vi "Arm - In Position Detector.vi"(6 "Angle Tolerance (+/-)":dbl=2.0 format="%#_13g", 8 "error in (no error)":errorcluster, 10 "Set Angle":dbl, 11 "AIDeviceRef":T1={"DevStatus"={"status"=FALSE, "code"=0, "source"=""}, "Analog Channel"=enum."Invalid"}) -> (0 "error out":errorcluster, 1 "In Position":bool, 2 "Current Angle":dbl, 4 "LED Control (Blink / On)":bool)   [LabVIEW 2015]
uses:
  <vilib>/Rock Robotics/WPI/AnalogChannel/WPI_AnalogChannelDevRef.ctl
  <vilib>/Rock Robotics/SystemInterfaces/AI/FPGA_AIChannel.ctl
  Global Variables.vi
panel:
  out "Voltage":dbl
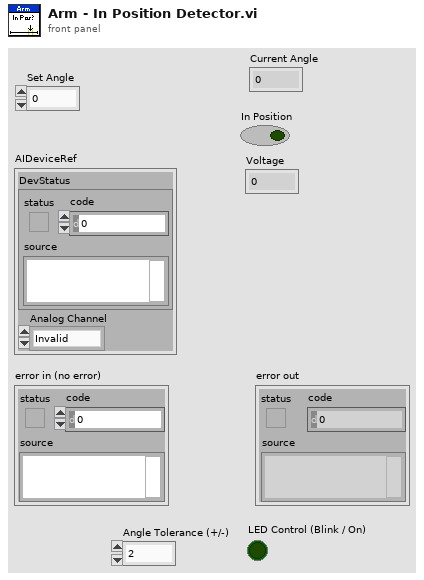
[diagram p1: front panel]
types:
  T1 = typedef "WPI_AnalogChannelDevRef.ctl" = cluster{"DevStatus":errorcluster, "Analog Channel":T2}
  T2 = typedef "FPGA_AIChannel.ctl" = enum8{"AI 0", "AI 1", "AI 2", "AI 3", "AI MXP 0", "AI MXP 1", "AI MXP 2", "AI MXP 3", "Invalid"}
  T3 = typedef "Robot Parameters.ctl" = cluster{"Robot Drive Parameters":cluster{"Teleop Drive Mode":enum16{"Split Axis Arcade", "Arcade Drive", "Tank Drive"}, "Drive PID Gains":cluster{"GRIP - Centering":cluster{"proportional gain (Kc)":dbl, "integral time (Ti, min)":dbl, "derivative time (Td, min)":dbl}, "GRIP - Area":cluster{"proportional gain (Kc)":dbl, "integral time (Ti, min)":dbl, "derivative time (Td, min)":dbl}, "Encoder":cluster{"proportional gain (Kc)":dbl, "integral time (Ti, min)":dbl, "derivative time (Td, min)":dbl}, "IMU - Spin":cluster{"proportional gain (Kc)":dbl, "integral time (Ti, min)":dbl, "derivative time (Td, min)":dbl}}}, "Shooter Parameters":cluster{"Open Claw Delay":u32, "Shoot Delay":u32, "Pressure Threshold for shooting":dbl}, "Arm Parameters":cluster{"PID gains":cluster{"proportional gain (Kc)":dbl, "integral time (Ti, min)":dbl, "derivative time (Td, min)":dbl}, "Arm Max Angle":dbl, "Arm Min Angle":dbl, "Default Angle":dbl, "Shoot Batter Angle":dbl, "Shoot Close Angle":dbl, "Shoot Far Angle":dbl, "Human Player Load Angle":dbl, "Low Bar / Goal Angle":dbl, "Arm Position Sensor Map":cluster{"Input Low (V)":dbl, "Input High (V)":dbl, "Output Low (Degree)":dbl, "Output High (Degree)":dbl}}, "Intake Parameters":cluster{"Suck In Speed":dbl, "Spit Out Speed":dbl}}
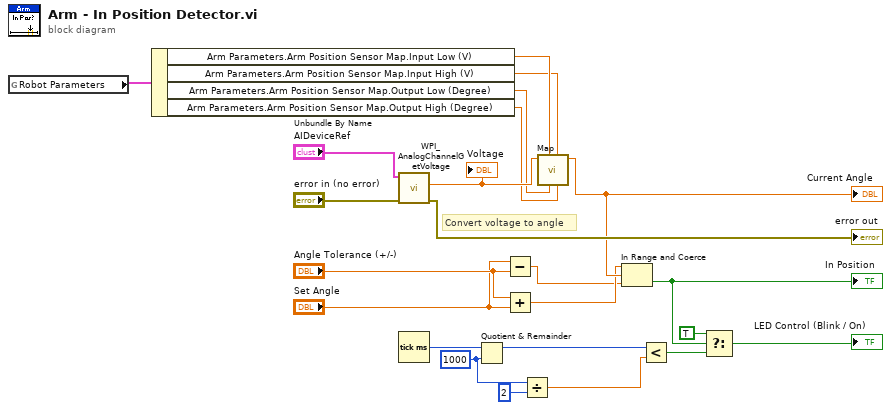
[diagram p0: block diagram]
diagram:
  w12 = u32 1000 ("y")
  # "Convert voltage to angle"
  n1 = global read "Global Variables.vi" "Robot Parameters"() -> (w7:T3)
  n2 = Unbundle By Name(w7) -> ("Arm Parameters.Arm Position Sensor Map.Input Low (V)"=w6:dbl, "Arm Parameters.Arm Position Sensor Map.Input High (V)"=w5:dbl, "Arm Parameters.Arm Position Sensor Map.Output Low (Degree)"=w4:dbl, "Arm Parameters.Arm Position Sensor Map.Output High (Degree)"=w3:dbl)
  n3 = call <vilib>:"WPI_AnalogChannelGetVoltage.vi"("error in (no error)"="error in (no error)", "AIDeviceRef"="AIDeviceRef") -> ("error out"=→"error out":errorcluster, "Voltage"=w9:dbl)  [unwired: 7 in, 1 out]
  "Voltage" <- w9
  n4 = Tick Count (ms)() -> (millisecond timer value=w19:u32)
  n5 = Quotient & Remainder(x=w19, y=w12) -> (x-y*floor(x/y)=w20:u32)  [unwired: 1 out]
  n6 = Subtract(x="Set Angle", y="Angle Tolerance (+/-)") -> (x-y=w1:dbl)
  n7 = Add(x="Angle Tolerance (+/-)", y="Set Angle") -> (x+y=w2:dbl)
  n8 = Divide(x=w12, y=u32 2) -> (x/y=w10:dbl)
  n9 = call "Map.vi"("Output High"=w3, "Input High"=w5, "Output Low"=w4, "Input Low"=w6, "Input"=w9) -> ("Output"=w8:dbl)  [unwired: 6 in]
  "Current Angle" <- w8
  n10 = In Range and Coerce(upper limit=w2, x=w8, lower limit=w1) -> (In Range?=w22:bool)  [unwired: 1 out]
  "In Position" <- w22
  n11 = Less?(x=w20, y=w10) -> (x < y?=w21:bool)
  n12 = Select(t=TRUE, s=w22, f=w21) -> (s? t:f=→"LED Control (Blink / On)":bool)
